vi "RSP_FAT_GENERIC_Command.vi"(0 "Error In":errorcluster, 1 "Response":u8[](array[numeric]) format="%x") -> (2 "Status":bool, 3 "Error Out":errorcluster, 4 "Generic_Mimic_Data":T1)   [LabVIEW 2014]
uses:
  MIMIC_ResponseCluster.ctl
panel:
  # "FAT GENERIC Response:"
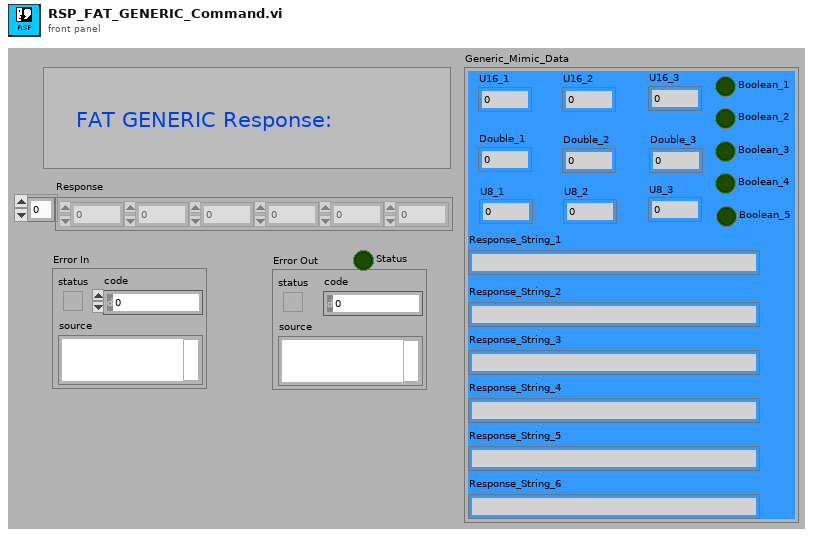
[diagram p1: front panel]
types:
  T1 = typedef "MIMIC_ResponseCluster.ctl" = cluster{"Response_String_1":string, "Response_String_2":string, "Response_String_3":string, "Response_String_4":string, "Response_String_5":string, "Response_String_6":string, "U16_1":u16, "Boolean_1":bool, "Boolean_2":bool, "Boolean_3":bool, "Boolean_4":bool, "Boolean_5":bool, "U16_2":u16, "U16_3":u16, "Double_1":dbl, "Double_2":dbl, "Double_3":dbl, "U8_1":dbl, "U8_2":dbl, "U8_3":dbl}
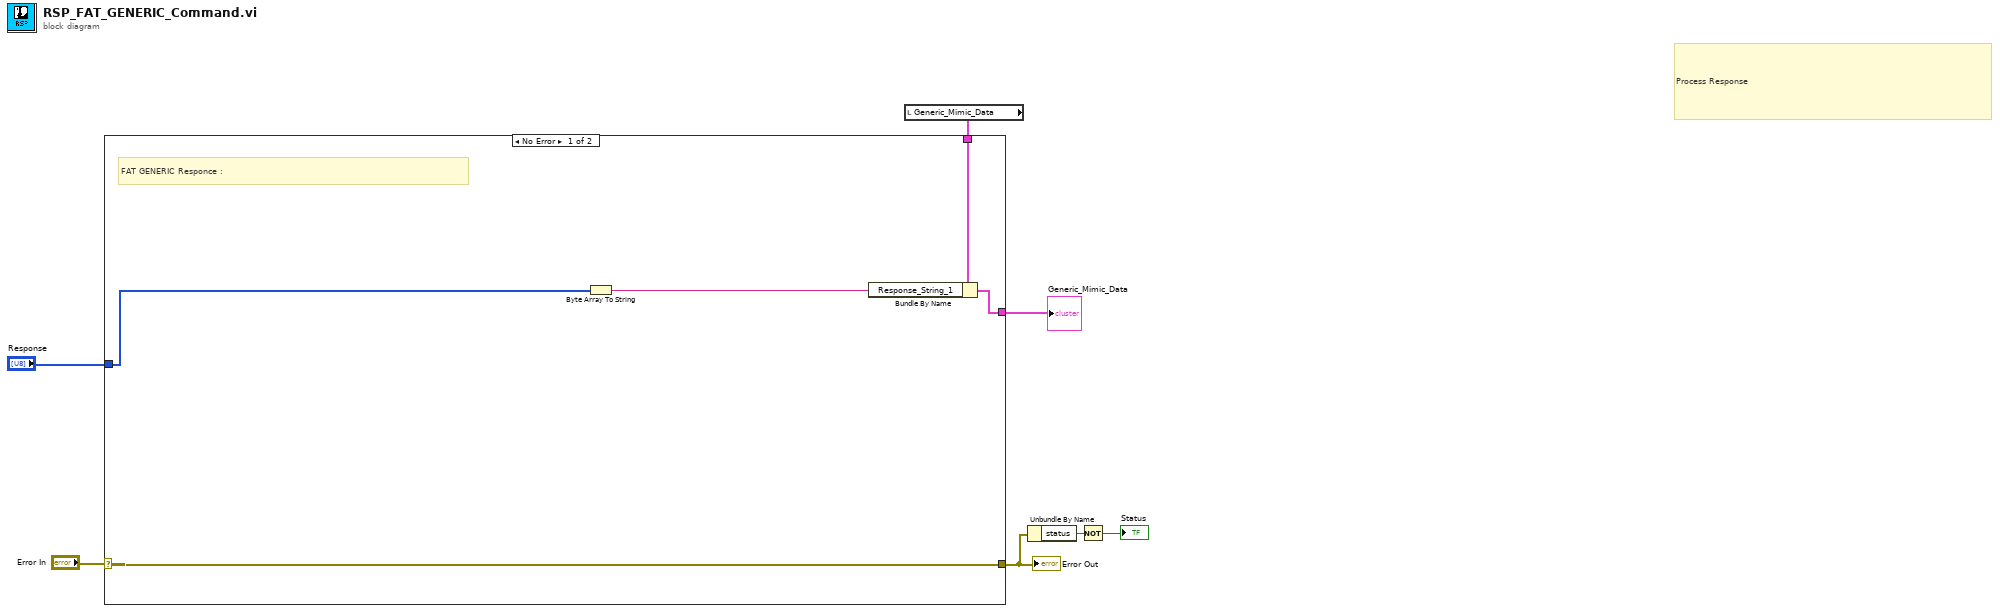
[diagram p0: block diagram]
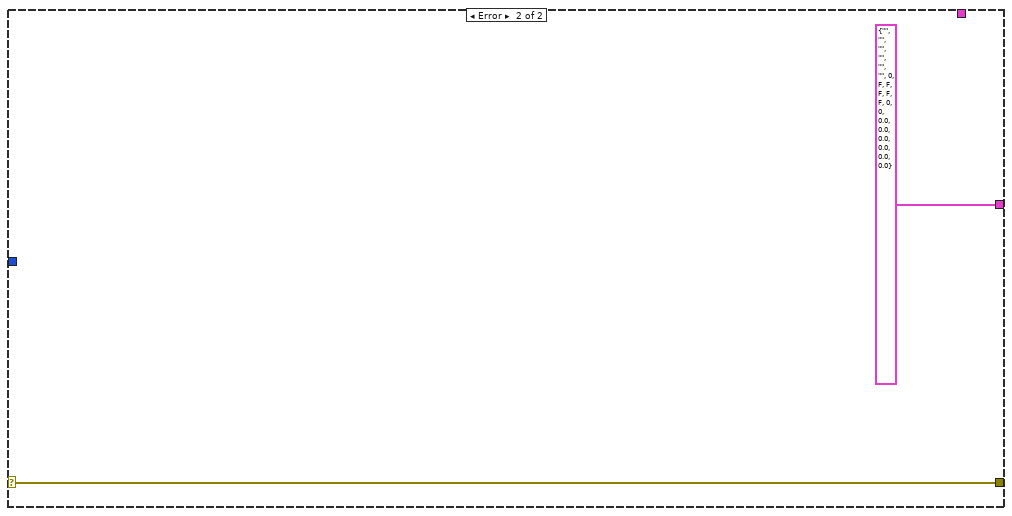
[diagram p2: hidden frame]
diagram:
  # "Process Response"
  n1 = local read "Generic_Mimic_Data"() -> (w2:T1)
  n2 = case shown="No Error" "Error In" {
    selector: "Error In" -> [w12 w14]
    tunnel: [w12 w14] -> w6
    tunnel: "Response" -> [w8 _]
    tunnel: w2 -> [w11 _]
    tunnel: [w10 T1 {"Response_String_1"="", "Response_String_2"="", "Response_String_3"="", "Response_String_4"="", "Response_String_5"="", "Response_String_6"="", "U16_1"=0, "Boolean_1"=FALSE, "Boolean_2"=FALSE, "Boolean_3"=FALSE, "Boolean_4"=FALSE, "Boolean_5"=FALSE, "U16_2"=0, "U16_3"=0, "Double_1"=0.0, "Double_2"=0.0, "Double_3"=0.0, "U8_1"=0.0, "U8_2"=0.0, "U8_3"=0.0} ("Generic_Mimic_Data")] -> w1
    frame No Error {
      # "FAT GENERIC Responce :"
      n3 = Byte Array To String(unsigned byte array=w8) -> (string=w9:string)
      n4 = Bundle By Name(cluster=w11, "Response_String_1"=w9) -> (w10:T1)
    }
    frame Error {
    }
  }
  "Error Out" <- w6
  "Generic_Mimic_Data" <- w1
  n5 = Unbundle By Name(w6) -> ("status"=w5:bool)
  n6 = Not(x=w5) -> (.not. x?=→"Status":bool)
